vi "ReadCurrentMeters.vi"(8 "Error In":errorcluster, 10 "Number of 6485":i32, 11 "Current Meters In":refnum<visa-resource-name>[](array[refnum])) -> (0 "Error Out":errorcluster, 2 "Current Meter Data":T1, 3 "Current Meters Out":refnum<visa-resource-name>[](array[refnum]))   [LabVIEW 2012]
uses:
  CurrentMeterData.ctl
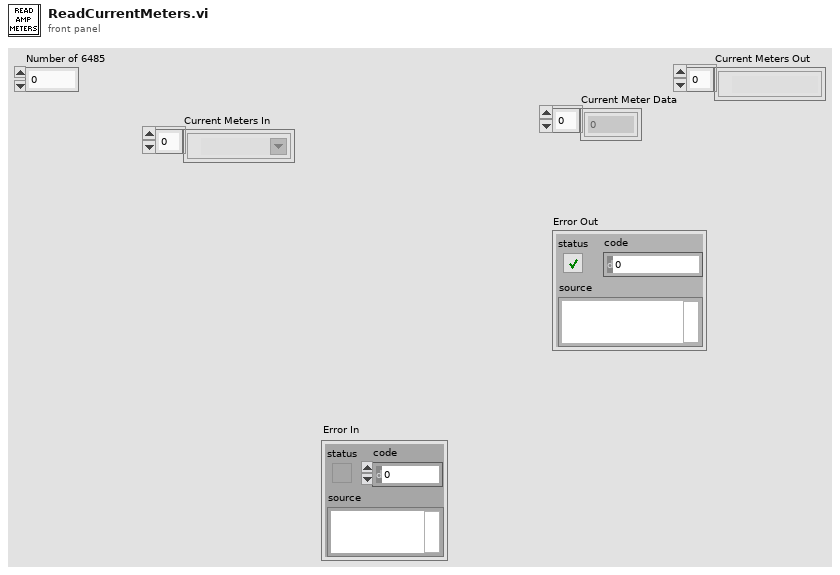
[diagram p1: front panel]
types:
  T1 = typedef "CurrentMeterData.ctl" = dbl[]
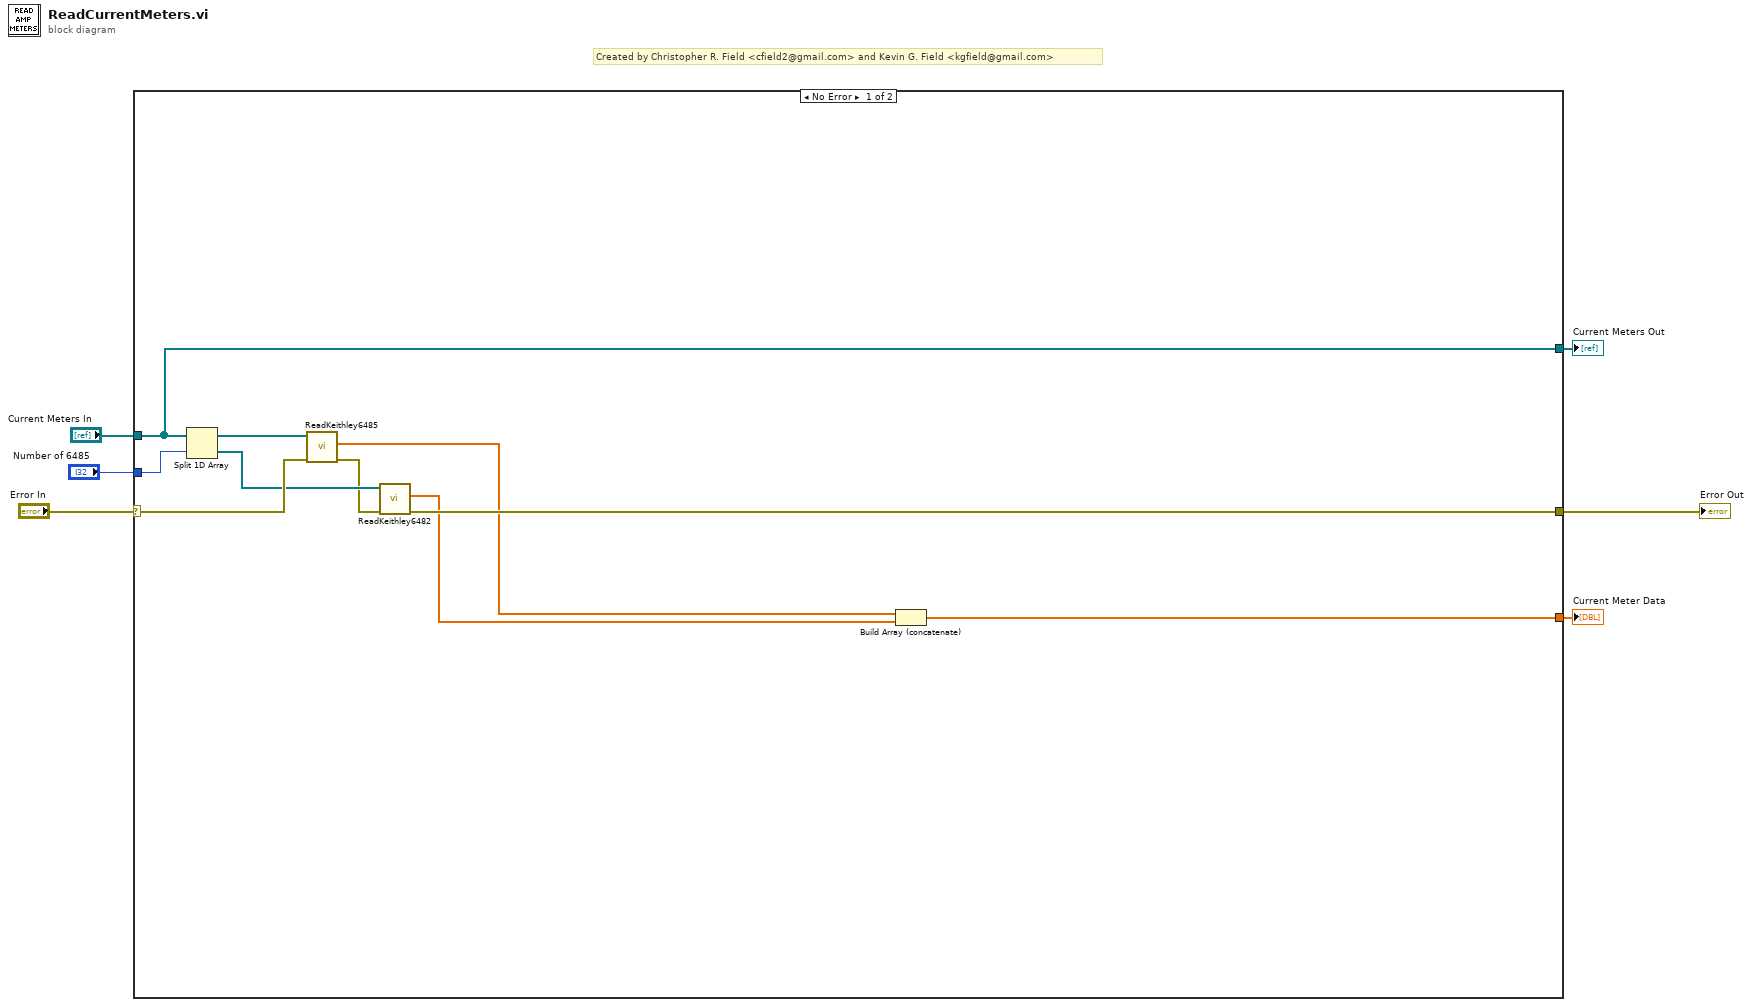
[diagram p0: block diagram]
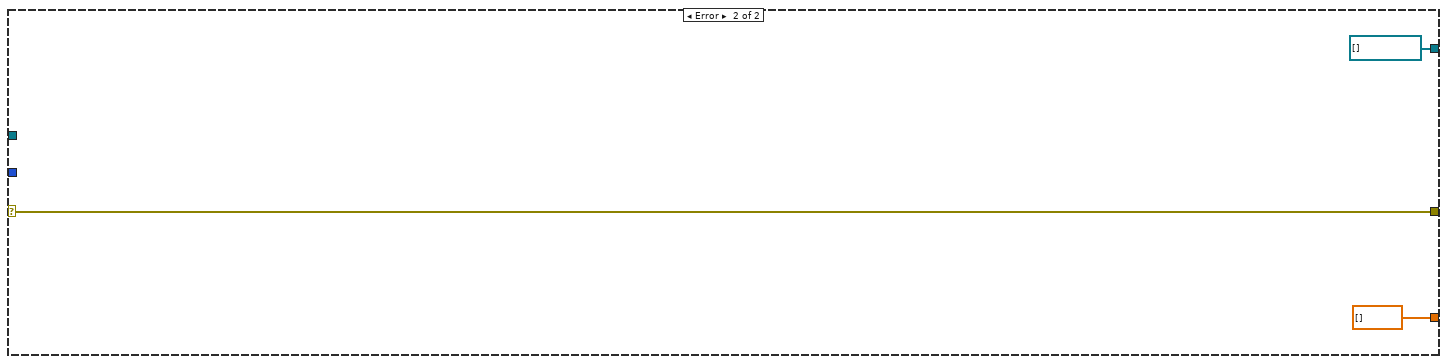
[diagram p2: hidden frame]
diagram:
  # "Created by Christopher R. Field <cfield2@gmail.com> and Kevin G. Field <kgfield@gmail.com>"
  n1 = case shown="No Error" "Error In" {
    selector: "Error In" -> [w14 w19]
    tunnel: "Current Meters In" -> [w10 _]
    tunnel: [w11 w19] -> w4
    tunnel: [w7 T1 [] ("Current Meter Data")] -> w3
    tunnel: "Number of 6485" -> [w16 _]
    tunnel: [w10 refnum<visa-resource-name>[] [] ("Current Meters In")] -> w1
    frame No Error {
      n2 = Split 1D Array(array=w10, index=w16) -> (first subarray=w15:refnum<visa-resource-name>[], second subarray=w13:refnum<visa-resource-name>[])
      n3 = call "ReadKeithley6485.vi"("Error In"=w14, "Keithley 6485 In"=w15) -> ("Error Out"=w12:errorcluster, "Data"=w9:dbl[])  [unwired: 7 in, 1 out]
      n4 = call "ReadKeithley6482.vi"("Error In"=w12, "Keithley 6482 In"=w13) -> ("Error Out"=w11:errorcluster, "Data"=w8:dbl[])  [unwired: 7 in, 1 out]
      n5 = Build Array (concatenate)(w9, w8) -> (w7:dbl[])
    }
    frame Error {
    }
  }
  "Error Out" <- w4
  "Current Meter Data" <- w3
  "Current Meters Out" <- w1
